vi "Lang Set Frame w.vi"(8 "error in (no error)":errorcluster, 10 "w":T1, 11 "LF2R IDE in":refnum<class "Main Panel.lvclass">) -> (0 "error out":errorcluster, 3 "LF2R IDE out":refnum<class "Main Panel.lvclass">)   [LabVIEW 2018, in "Main Panel.lvlib" / "Main Panel.lvclass"]
uses:
  Main Panel.lvclass
  Framework/Framework/Const Lang MainWnd Frame w.ctl
  Framework/Framework/Const Lang Property.ctl
  Main Panel.lvclass/Main Panel.ctl
  Framework/Framework/Framework.lvclass
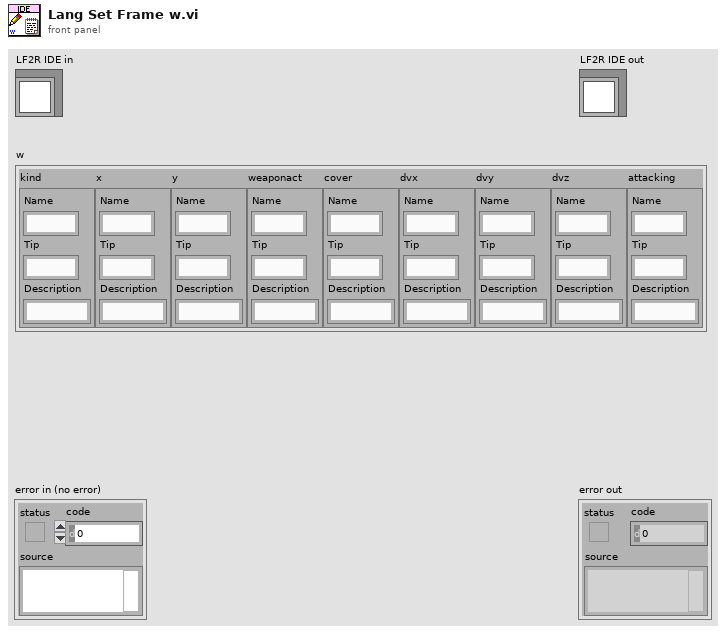
[diagram p1: front panel]
types:
  T1 = typedef "Framework.lvlib/Framework.lvclass/Const Lang MainWnd Frame w.ctl" = cluster{"kind":T2, "x":T2, "y":T2, "weaponact":T2, "cover":T2, "dvx":T2, "dvy":T2, "dvz":T2, "attacking":T2}
  T2 = typedef "Framework.lvlib/Framework.lvclass/Const Lang Property.ctl" = cluster{"Name":string, "Tip":string, "Description":string}
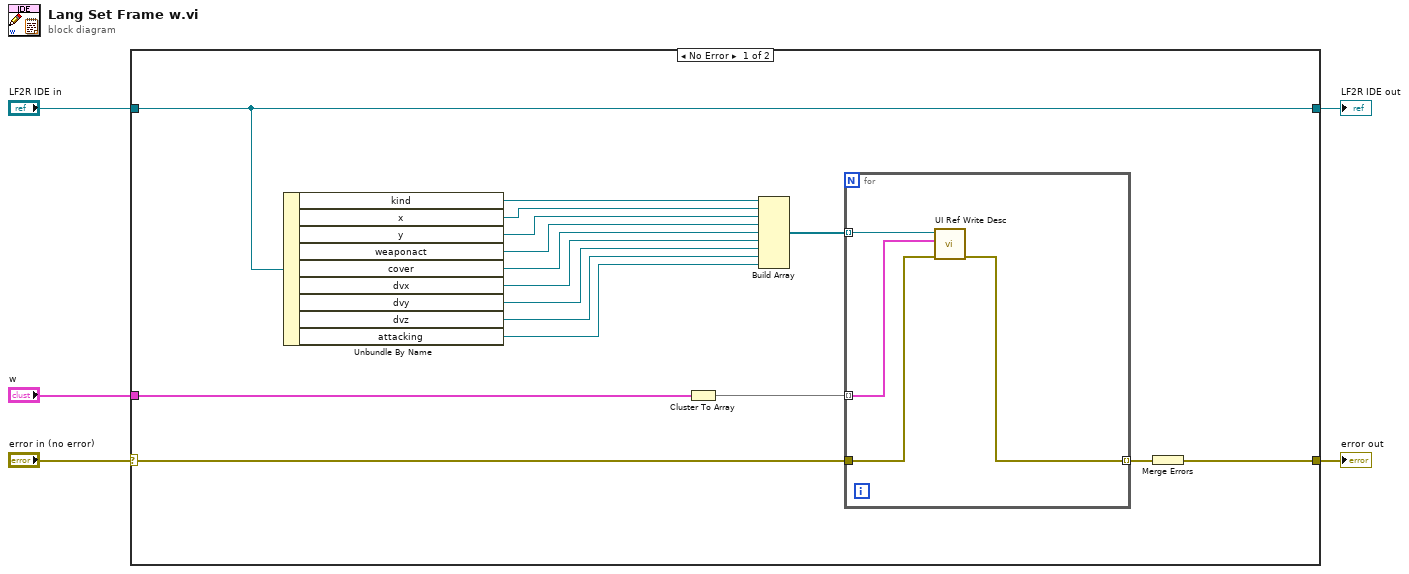
[diagram p0: block diagram]
diagram:
  n1 = case shown="No Error" "error in (no error)" {
    selector: "error in (no error)" -> [w17 w27]
    tunnel: [w15 w27] -> w4
    tunnel: [w21 w26] -> w2
    tunnel: "LF2R IDE in" -> [w21 w26]
    tunnel: "w" -> [w19 _]
    frame No Error {
      n2 = Unbundle By Name(w21) -> ("kind"=w14:refnum<vi>, "x"=w13:refnum<vi>, "y"=w12:refnum<vi>, "weaponact"=w11:refnum<vi>, "cover"=w9:refnum<vi>, "dvx"=w10:refnum<vi>, "dvy"=w8:refnum<vi>, "dvz"=w7:refnum<vi>, "attacking"=w6:refnum<vi>)
      n3 = Cluster To Array(cluster=w19) -> (array=w18:T2[])
      n4 = Build Array(w14, w13, w12, w11, w9, w10, w8, w7, w6) -> (w20:refnum<vi>[])
      n5 = for {
        tunnel: w20 -> [w22] mode=indexing
        tunnel: w18 -> [w25] mode=indexing
        tunnel: w17 -> [w24]
        tunnel: [w23] -> w16 mode=indexing
        n6 = call "UI Ref Write Desc.vi"("error in (no error)"=w24, "UI Property"=w25, "UI Ref"=w22) -> ("error out"=w23:errorcluster)  [unwired: 8 in]
      }
      n7 = Merge Errors(w16) -> (w15:errorcluster)
    }
    frame Error {
    }
  }
  "error out" <- w4
  "LF2R IDE out" <- w2
